vi "Airmar Interpret NMEA Sentence.vi"(11 "NMEA Sentence":string) -> ()   [LabVIEW 2013]
doc: "Interprets the NMEA 0813 sentences that we are using from our Airmar PB200 WeatherStation sensor.\nBy Jaime McCandless\nTODO: finish implementing NMEA sentences"
uses:
  Data/TypeDefs/UTM Location.ctl
  Data/TypeDefs/Notifiers.ctl
  Data/TypeDefs/GPS Sensor Status.ctl
  Data/TypeDefs/Sail Set Suggestions.ctl
  Data/TypeDefs/Rudder Set Suggestions.ctl
  <vilib>/regexp/Match Regular Expression.xnode
panel:
  in  "NotifierReff 2":T1
  in  "UTC Time Zone":i32=-5
  in  "Tab Control":T2(tab)
  out "GPS (GGA) Data":T3
  out "GPS (GLL) Data":T4
  out "GPGSA Data":T5
  out "UTC Time":timestamp
  out "Local Time":timestamp
  out "Lattitude (ddmm.mmmm)":dbl format="%_8g"
  out "Lattitude North/South":string
  out "Longitude (ddmm.mmmm)":dbl format="%_8g"
  out "Longitude East/West":string
  out "Speed over ground (knots)":dbl format="%_3g"
  out "Course over ground (degrees)":dbl format="%_4g"
  out "Magnetic Variation (degrees)":dbl format="%_4g"
  out "Variation East/West":string
  out "GPS (RMC) Data":T6 {"Course over ground (degrees)" format="%#.6g"; "Speed over ground (knots)" format="%#.6g"; "Magnetic Variation (degrees)" format="%#.6g"; "Longitude (ddmm.mmmm)" format="%#.6g"; "Lattitude (ddmm.mmmm)" format="%#.6g"}
  out "GPS Data Valid?":bool
  out "Robot UTM Location":T7 {"North" format="%#_10f"; "East" format="%#_8f"}
  out "GPS (VTG) Data":T8
  out "Heading":dbl
  out "Turn (ROT) Data":T9
  out "Meteorological Data":T10
  out "Relative wind direction":cluster{dbl, "Filtered Value Out":dbl}(graph)
  out "Wind (MWV) Data, Theoretical":T11
  out "Wind (MWV) Data, Relative":T11
  out "Transducer (XDR) B Data":cluster{"Pitch (deg)":dbl, "Roll (deg)":dbl}
  out "Transducer (XDR) A Data":T12
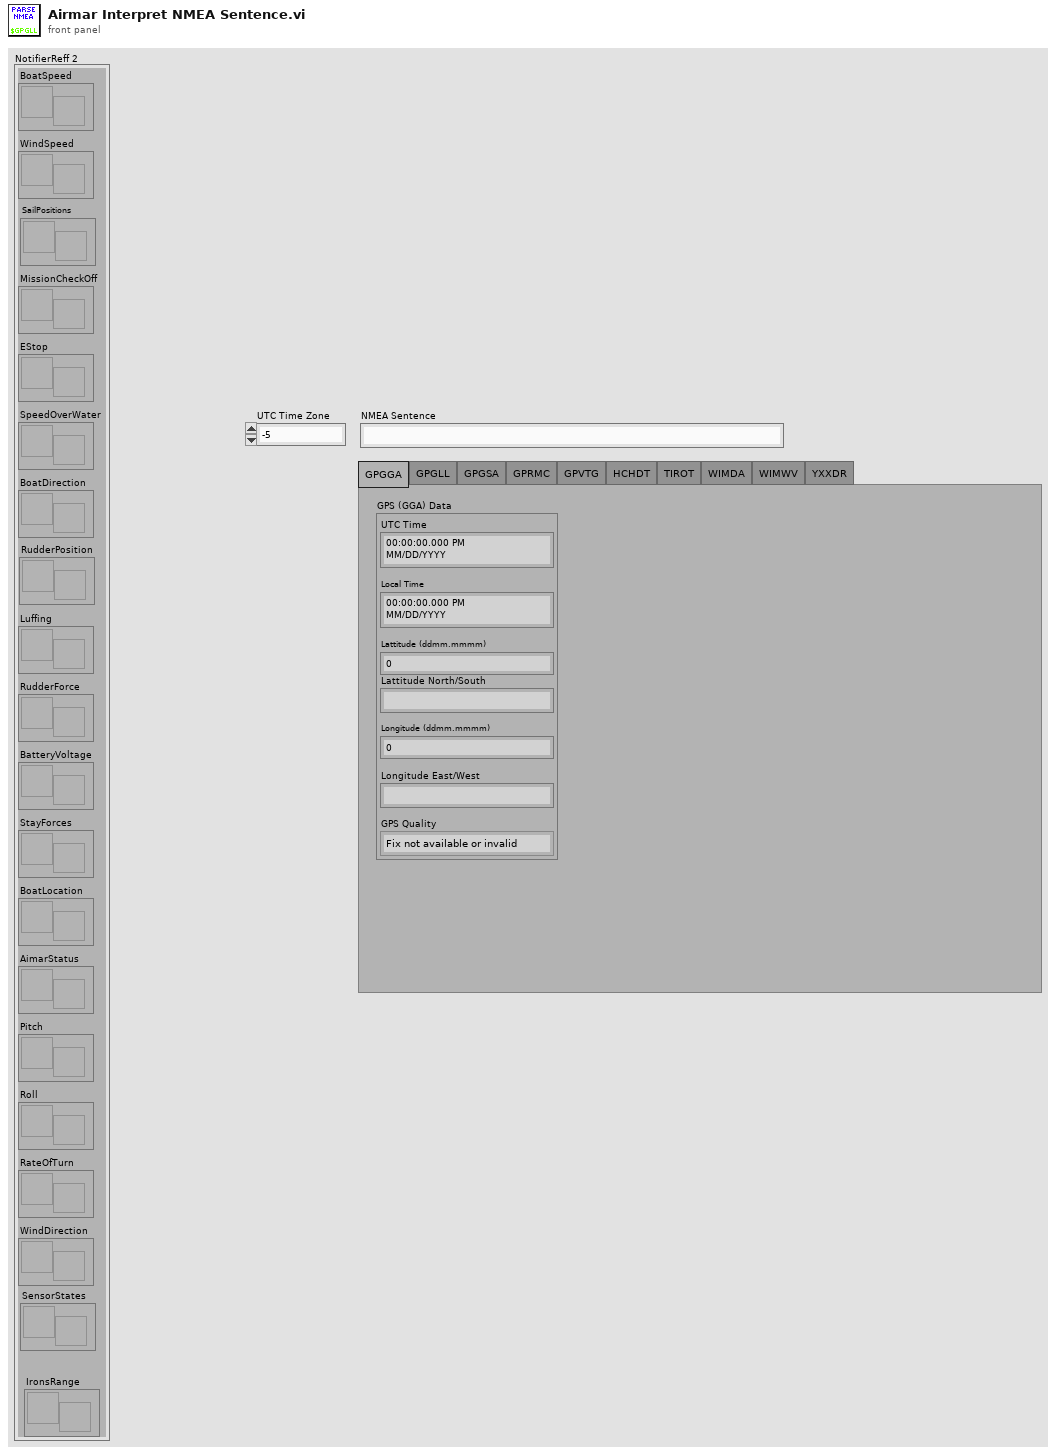
[diagram p1: front panel]
types:
  T1 = typedef "Notifiers.ctl" = cluster{"BoatSpeed":refnum<notifier>, "WindSpeed":refnum<notifier>, "MissionCheckOff":refnum<notifier>, "EStop":refnum<notifier>, "SpeedOverWater":refnum<notifier>, "BoatDirection":refnum<notifier>, "Luffing":refnum<notifier>, "RudderForce":refnum<notifier>, "BatteryVoltage":refnum<notifier>, "StayForces":refnum<notifier>, "BoatLocation":refnum<notifier>, "AimarStatus":refnum<notifier>, "Pitch":refnum<notifier>, "Roll":refnum<notifier>, "RateOfTurn":refnum<notifier>, "WindDirection":refnum<notifier>, "SailPositions":refnum<notifier>, "RudderPosition":refnum<notifier>, "SensorStates":refnum<notifier>, "IronsRange":refnum<notifier>}
  T2 = enum32{"GPGGA", "GPGLL", "GPGSA", "GPRMC", "GPVTG", "HCHDT", "TIROT", "WIMDA", "WIMWV", "YXXDR"}
  T3 = cluster{"UTC Time":timestamp, "Local Time":timestamp, "Lattitude (ddmm.mmmm)":dbl, "Lattitude North/South":string, "Longitude (ddmm.mmmm)":dbl, "Longitude East/West":string, "GPS Quality":enum16{"Fix not available or invalid", "GPS SPS Mode, fix valid", "Differential GPS, SPS Mode, fix valid", "GPS PPS Mode, fix valid", "Real Time Kinematic (RTK)", "Float RTK", "Estimated (dead reckoning) Mode", "Manual Input Mode", "Simulator Mode"}}
  T4 = cluster{"UTC Time":timestamp, "Local Time":timestamp, "Lattitude (ddmm.mmmm)":dbl, "Lattitude North/South":string, "Longitude (ddmm.mmmm)":dbl, "Longitude East/West":string, "GPS Mode":string, "GPS Data Valid?":bool}
  T5 = cluster{"Mode":string, "Fix Strength":i32, "Satellite IDs":i32[], "PDOP":dbl, "HDOP":dbl, "VDOP":dbl}
  T6 = cluster{"UTC Time":timestamp, "Local Time":timestamp, "Lattitude (ddmm.mmmm)":dbl, "Lattitude North/South":string, "Longitude (ddmm.mmmm)":dbl, "Longitude East/West":string, "Magnetic Variation (degrees)":dbl, "Variation East/West":string, "Speed over ground (knots)":dbl, "Course over ground (degrees)":dbl}
  T7 = typedef "UTM Location.ctl" = cluster{"UTM Zone":dbl, "Hemisphere":enum16{"North", "South"}, "East":dbl, "North":dbl}
  T8 = cluster{"Course Over Ground (True)":dbl, "Course Over Ground (Magnetic)":dbl, "Speed Over Ground (Knots)":dbl, "Speed Over Ground (km/hr)":dbl, "GPS Mode":string}
  T9 = cluster{"Rate of Turn (deg/min)":dbl, "Turn Rotation Data Valid?":bool}
  T10 = cluster{"Barometric Pressure (inches of mercury)":dbl, "Barometric Pressure (bars)":dbl, "Air temperature (degC)":dbl, "Relative humidity (%)":dbl, "Wind direction, True (deg)":dbl, "Wind direction, Magnetic (deg)":dbl, "Wind speed (knots)":dbl, "Wind speed (m/s)":dbl}
  T11 = cluster{"Angle relative to boat (deg)":dbl, "Wind Data Valid?":bool, "Wind speed (knots)":dbl, "True (T) or Relative (R)":string}
  T12 = cluster{"Calc. Relative Wind Chill (degC)":dbl, "Calc. Theoretical Wind Chill (degC)":dbl, "Calc. Heat Index (degC)":dbl, "Meas. Barometric Pressure (bars)":dbl}
  T13 = typedef "GPS Sensor Status.ctl" = cluster{"Sensor Connected":bool, "Sensor OK":bool, "GPS Lock":bool, "Sensor Initialized":bool}
  T14 = cluster{"second":i32, "minute":i32, "hour":i32, "day of month":i32, "month":i32, "year":i32, "day of week":i32, "day of year":i32, "is DST":i32}
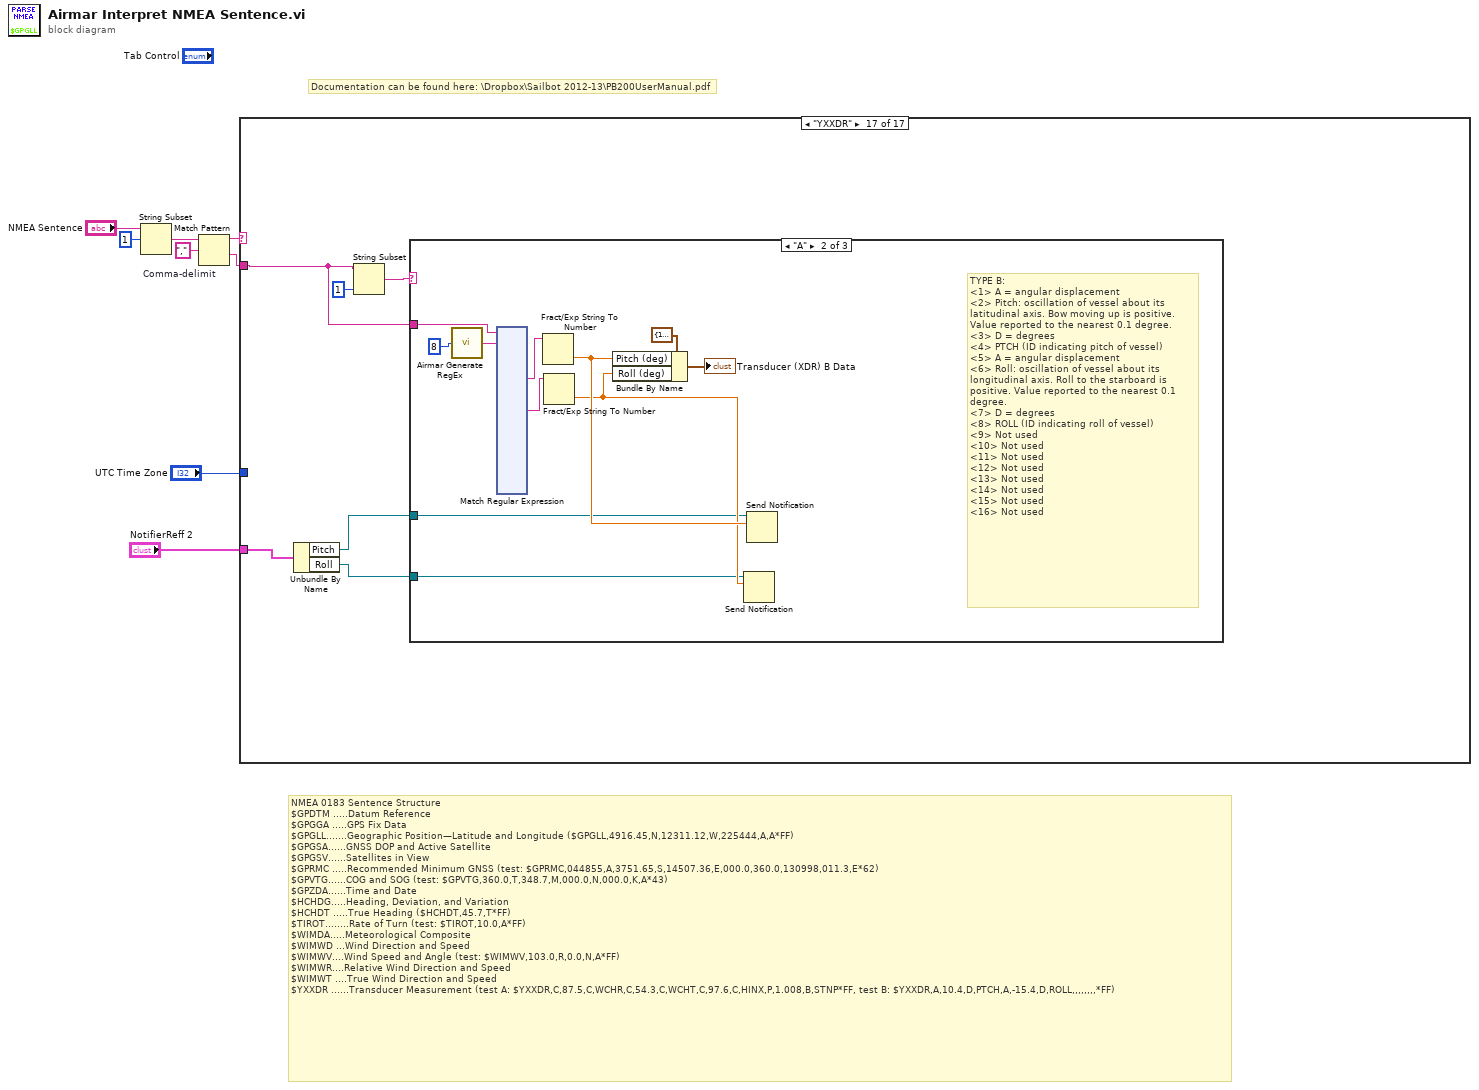
[diagram p0: block diagram]
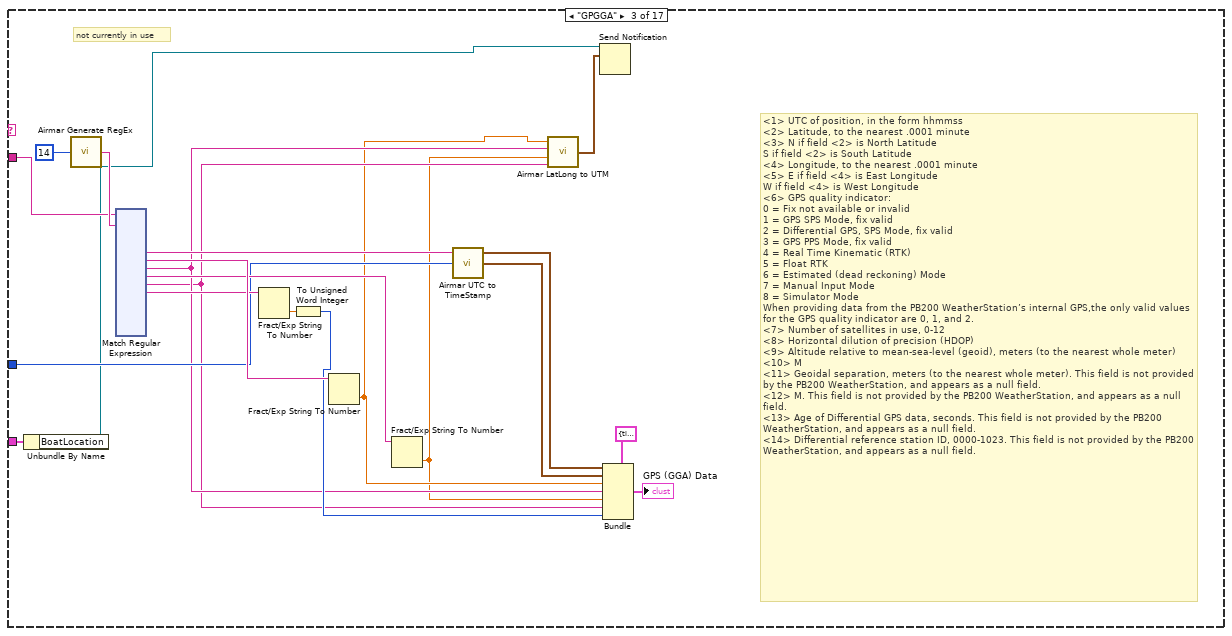
[diagram p4: hidden frame]
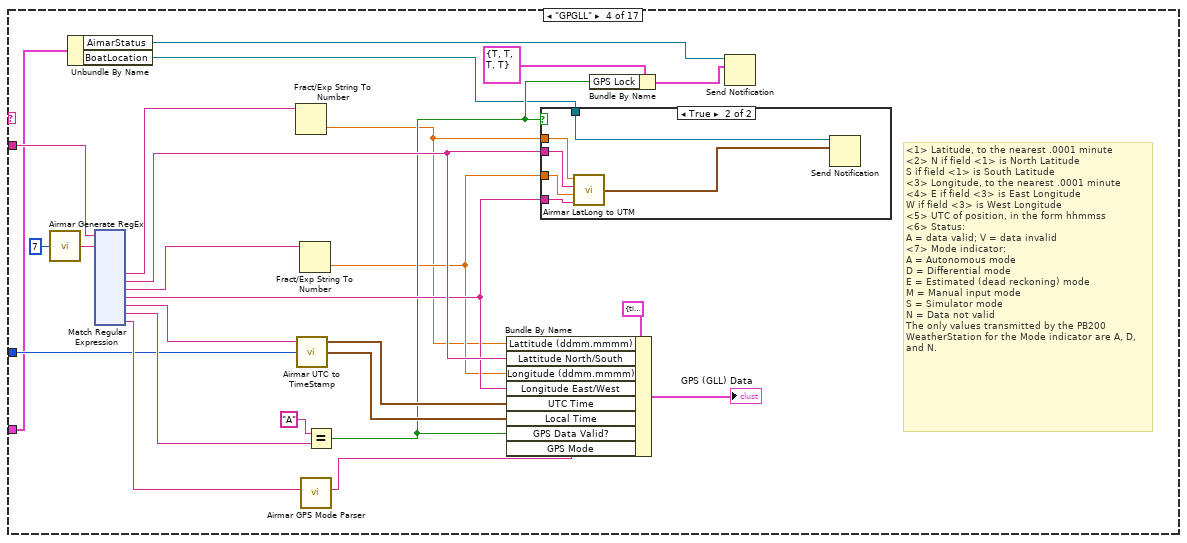
[diagram p5: hidden frame]
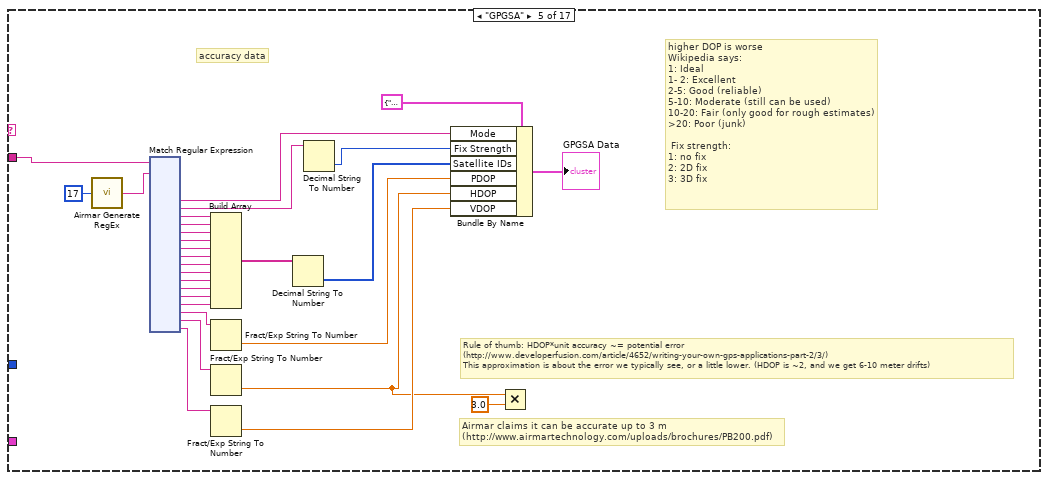
[diagram p7: hidden frame]
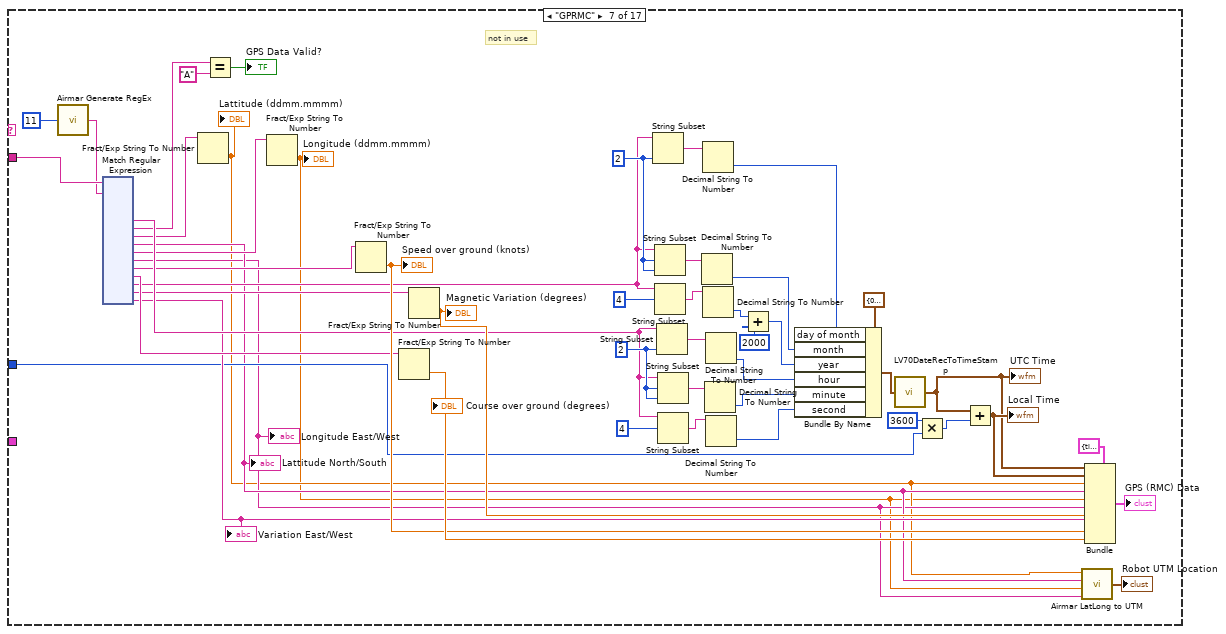
[diagram p9: hidden frame]
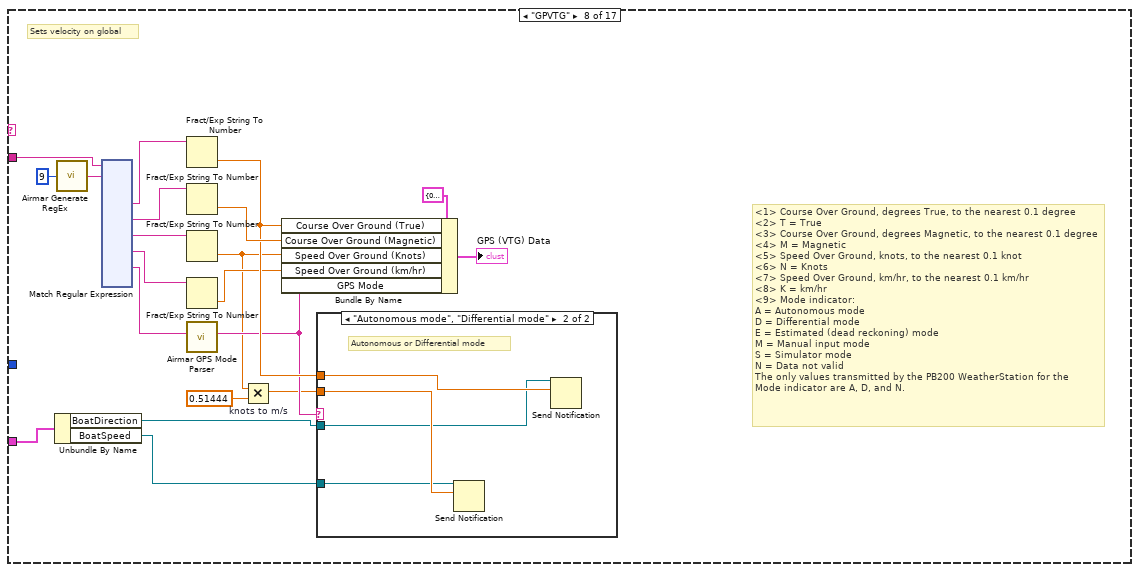
[diagram p10: hidden frame]
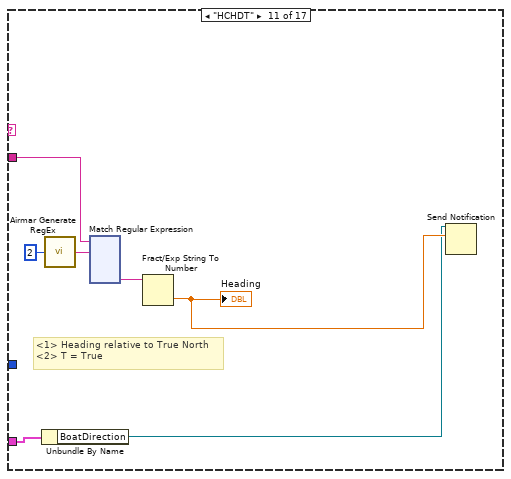
[diagram p14: hidden frame]
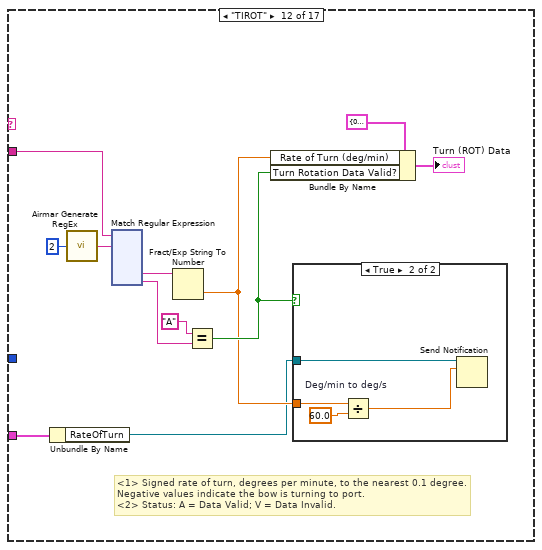
[diagram p15: hidden frame]
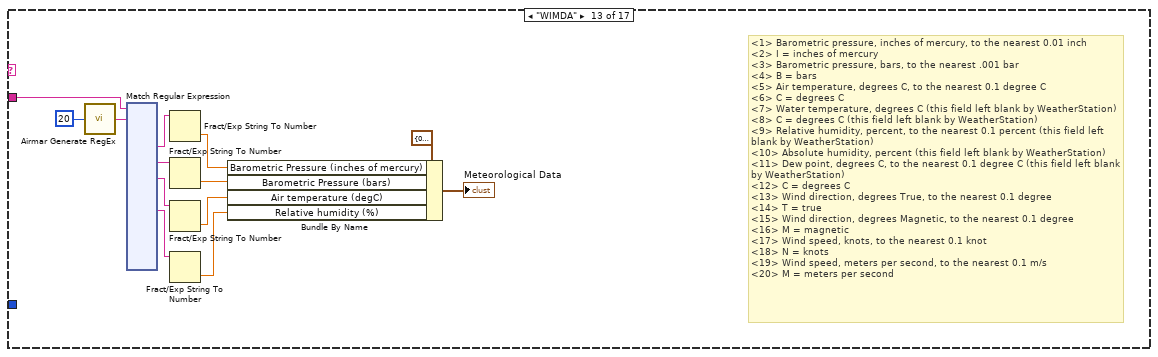
[diagram p17: hidden frame]
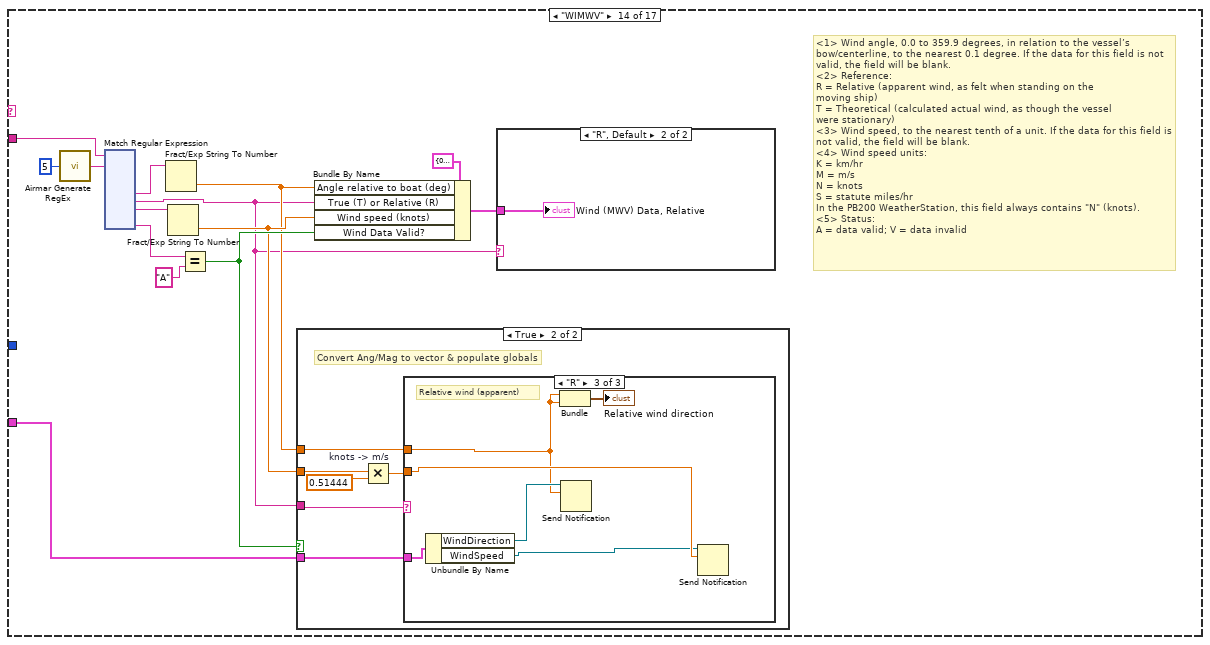
[diagram p18: hidden frame]
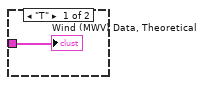
[diagram p19: hidden frame]
diagram:
  # "Documentation can be found here: \\Dropbox\\Sailbot 2012-13\\PB200UserManual.pdf"
  # "NMEA 0183 Sentence Structure\n$GPDTM .....Datum Reference\n$GPGGA .....GPS Fix Data\n$GPGLL.......Geographic Position—Latitude and Longitude ($GPGLL,4916.45,N,12311.12,W,225444,A,A*FF)\n$GPGSA......GNSS DOP and Active Satellite\n$GPGSV......Satellites in View\n$GPRMC .....Recommended Minimum GNSS (test: $GPRMC,044855,A,3751.65,S,14507.36,E,000.0,360.0,130998,011.3,E*62)\n$GPVTG......COG and SOG (test: $GPVTG,360.0,T,348.7,M,000.0,N,000.0,K,A*43)\n$GPZDA......Time and Date\n$HCHDG.....Heading, Deviation, and Variation\n$HCHDT .....True Heading ($HCHDT,45.7,T*FF)\n$TIROT........Rate of Turn (test: $TIROT,10.0,A*FF)\n$WIMDA.....Meteorological Composite\n$WIMWD ...Wind Direction and Speed\n$WIMWV....Wind Speed and Angle (test: $WIMWV,103.0,R,0.0,N,A*FF)\n$WIMWR....Relative Wind Direction and Speed\n$WIMWT ....True Wind Direction and Speed\n$YXXDR ......Transducer Measurement (test A: $YXXDR,C,87.5,C,WCHR,C,54.3,C,WCHT,C,97.6,C,HINX,P,1.008,B,STNP*FF, test B: $YXXDR,A,10.4,D,PTCH,A,-15.4,D,ROLL,,,,,,,,*FF)"
  n1 = String Subset(string="NMEA Sentence", offset (0)=1) -> (substring=w5:string)  [unwired: 1 in]
  n2 = Match Pattern "Comma-delimit"(string=w5, regular expression=",") -> (before substring=w6:string, after substring=w7:string)  [unwired: 1 in, 2 out]
  n3 = case shown="\"YXXDR\"" w6 {
    tunnel: w7 -> [_ _ w27 w172 w331 _ w478 w650 _ _ w784 w908 w1040 w1180 _ _ w1319]
    tunnel: "UTC Time Zone" -> [_ _ w16 w164 _ _ w466 _ _ _ _ _ _ _ _ _ _]
    tunnel: "NotifierReff 2" -> [_ _ w12 w157 _ _ _ w635 _ _ w781 w901 _ w1171 _ _ w1318]
    frame "", Default {
    }
    frame "GPDTM" {
      # "unimplemented"
    }
    frame "GPGGA" {
      # "not currently in use"
      # "<1> UTC of position, in the form hhmmss\n<2> Latitude, to the nearest .0001 minute\n<3> N if field <2> is North Latitude\nS if field <2> is South Latitude\n<4> Longitude, to the nearest .0001 minute\n<5> E if field <4> is East Longitude\nW if field <4> is West Longitude\n<6> GPS quality indicator:\n0 = Fix not available or invalid\n1 = GPS SPS Mode, fix valid\n2 = Differential GPS, SPS Mode, fix valid\n3 = GPS PPS Mode, fix valid\n4 = Real Time Kinematic (RTK)\n5 = Float RTK\n6 = Estimated (dead reckoning) Mode\n7 = Manual Input Mode\n8 = Simulator Mode\nWhen providing data from the PB200 WeatherStation’s internal GPS,the only valid values for the GPS quality indicator are 0, 1, and 2.\n<7> Number of satellites in use, 0-12\n<8> Horizontal dilution of precision (HDOP)\n<9> Altitude relative to mean-sea-level (geoid), meters (to the nearest whole meter)\n<10> M\n<11> Geoidal separation, meters (to the nearest whole meter). This field is not provided by the PB200 WeatherStation, and appears as a null field.\n<12> M. This field is not provided by the PB200 WeatherStation, and appears as a null field.\n<13> Age of Differential GPS data, seconds. This field is not provided by the PB200 WeatherStation, and appears as a null field.\n<14> Differential reference station ID, 0000-1023. This field is not provided by the PB200 WeatherStation, and appears as a null field."
      n4 = Unbundle By Name(w12) -> ("BoatLocation"=w11:refnum<notifier>)
      n5 = call "Airmar Generate RegEx.vi"("# Datums"=14) -> ("RegEx"=w28:string)
      n6 = xnode "Match Regular Expression"("input string"=w27, "regular expression"=w28) -> ("submatch 1"=w19:string, "submatch 2"=w25:string, "submatch 3"=w15:string, "submatch 4"=w24:string, "submatch 5"=w14:string, "submatch 6"=w23:string)  [unwired: 4 in, 10 out]
      n7 = Fract/Exp String To Number(string=w23) -> (number=w22:dbl)  [unwired: 3 in, 1 out]
      n8 = To Unsigned Word Integer(number=w22) -> (unsigned 16bit integer=w21:u16)
      n9 = Fract/Exp String To Number(string=w25) -> (number=w10:dbl)  [unwired: 3 in, 1 out]
      n10 = Fract/Exp String To Number(string=w24) -> (number=w9:dbl)  [unwired: 3 in, 1 out]
      n11 = call "Airmar UTC to TimeStamp.vi"("UTC Time Zone in"=w16, "UTC (hhmmss)"=w19) -> ("Local Time"=w17:timestamp, "UTC Time"=w18:timestamp)  [unwired: 2 in]
      n12 = call "Airmar LatLong to UTM.vi"("East/West"=w14, "Longitude"=w9, "North/South"=w15, "Latitude"=w10) -> ("Robot UTM Location"=w13:T7)
      n13 = Send Notification(notification=w13, notifier=w11) -> ()  [unwired: 1 in, 2 out]
      n14 = Bundle(cluster=T3 {"UTC Time"=timestamp(0 s since 1904-01-01), "Local Time"=timestamp(0 s since 1904-01-01), "Lattitude (ddmm.mmmm)"=0.0, "Lattitude North/South"="", "Longitude (ddmm.mmmm)"=0.0, "Longitude East/West"="", "GPS Quality"=enum."GPS SPS Mode, fix valid"} ("Cluster"), "UTC Time"=w18, "Local Time"=w17, "Lattitude (ddmm.mmmm)"=w10, "Lattitude North/South"=w15, "Longitude (ddmm.mmmm)"=w9, "Longitude East/West"=w14, "GPS Quality"=w21) -> (→"GPS (GGA) Data":T3)
    }
    frame "GPGLL" {
      # "<1> Latitude, to the nearest .0001 minute\n<2> N if field <1> is North Latitude\nS if field <1> is South Latitude\n<3> Longitude, to the nearest .0001 minute\n<4> E if field <3> is East Longitude\nW if field <3> is West Longitude\n<5> UTC of position, in the form hhmmss\n<6> Status:\nA = data valid; V = data invalid\n<7> Mode indicator:\nA = Autonomous mode\nD = Differential mode\nE = Estimated (dead reckoning) mode\nM = Manual input mode\nS = Simulator mode\nN = Data not valid\nThe only values transmitted by the PB200 WeatherStation for the Mode indicator are A, D, and N."
      n15 = call "Airmar Generate RegEx.vi"("# Datums"=7) -> ("RegEx"=w176:string)
      n16 = Unbundle By Name(w157) -> ("AimarStatus"=w153:refnum<notifier>, "BoatLocation"=w156:refnum<notifier>)
      n17 = xnode "Match Regular Expression"("input string"=w172, "regular expression"=w176) -> ("submatch 1"=w175:string, "submatch 2"=w162:string, "submatch 3"=w174:string, "submatch 4"=w161:string, "submatch 5"=w171:string, "submatch 6"=w167:string, "submatch 7"=w173:string)  [unwired: 4 in, 5 out]
      n18 = Fract/Exp String To Number(string=w175) -> (number=w154:dbl)  [unwired: 3 in, 1 out]
      n19 = call "Airmar UTC to TimeStamp.vi"("UTC Time Zone in"=w164, "UTC (hhmmss)"=w171) -> ("Local Time"=w166:timestamp, "UTC Time"=w165:timestamp)  [unwired: 2 in]
      n20 = Fract/Exp String To Number(string=w174) -> (number=w155:dbl)  [unwired: 3 in, 1 out]
      n21 = call "Airmar GPS Mode Parser.vi"("GPS Mode (Char)"=w173) -> ("GPS Mode (Description)"=w169:string)  [unwired: 6 in]
      n22 = Equal?(x="A" ("y"), y=w167) -> (x = y?=w160:bool)
      n23 = Bundle By Name(cluster=T4 {"UTC Time"=timestamp(0 s since 1904-01-01), "Local Time"=timestamp(0 s since 1904-01-01), "Lattitude (ddmm.mmmm)"=0.0, "Lattitude North/South"="", "Longitude (ddmm.mmmm)"=0.0, "Longitude East/West"="", "GPS Mode"="", "GPS Data Valid?"=FALSE} ("Cluster"), "Lattitude (ddmm.mmmm)"=w154, "Lattitude North/South"=w162, "Longitude (ddmm.mmmm)"=w155, "Longitude East/West"=w161, "UTC Time"=w165, "Local Time"=w166, "GPS Data Valid?"=w160, "GPS Mode"=w169) -> (→"GPS (GLL) Data":T4)
      n24 = case shown="True" w160 {
        tunnel: w162 -> [_ w183]
        tunnel: w155 -> [_ w182]
        tunnel: w161 -> [_ w181]
        tunnel: w156 -> [_ w179]
        tunnel: w154 -> [_ w178]
        frame False {
        }
        frame True {
          n25 = call "Airmar LatLong to UTM.vi"("East/West"=w181, "Longitude"=w182, "North/South"=w183, "Latitude"=w178) -> ("Robot UTM Location"=w180:T7)
          n26 = Send Notification(notification=w180, notifier=w179) -> ()  [unwired: 1 in, 2 out]
        }
      }
      n27 = Bundle By Name(cluster=T13 {"Sensor Connected"=TRUE, "Sensor OK"=TRUE, "GPS Lock"=TRUE, "Sensor Initialized"=TRUE} ("input cluster"), "GPS Lock"=w160) -> (w158:T13)
      n28 = Send Notification(notification=w158, notifier=w153) -> ()  [unwired: 1 in, 2 out]
    }
    frame "GPGSA" {
      # "Airmar claims it can be accurate up to 3 m\n(http://www.airmartechnology.com/uploads/brochures/PB200.pdf)"
      # "Rule of thumb: HDOP*unit accuracy ~= potential error\n(http://www.developerfusion.com/article/4652/writing-your-own-gps-applications-part-2/3/)\nThis approximation is about the error we typically see, or a little lower. (HDOP is ~2, and we get 6-10 meter drifts)"
      # "higher DOP is worse\nWikipedia says:\n1: Ideal\n1- 2: Excellent\n2-5: Good (reliable)\n5-10: Moderate (still can be used)\n10-20: Fair (only good for rough estimates)\n>20: Poor (junk)\n\n Fix strength: \n1: no fix\n2: 2D fix\n3: 3D fix"
      # "accuracy data"
      n29 = call "Airmar Generate RegEx.vi"("# Datums"=17) -> ("RegEx"=w330:string)
      n30 = xnode "Match Regular Expression"("input string"=w331, "regular expression"=w330) -> ("submatch 1"=w327:string, "submatch 2"=w326:string, "submatch 3"=w324:string, "submatch 4"=w323:string, "submatch 5"=w322:string, "submatch 6"=w321:string, "submatch 7"=w320:string, "submatch 8"=w319:string, "submatch 9"=w318:string, "submatch 10"=w317:string, "submatch 11"=w316:string, "submatch 12"=w315:string, "submatch 13"=w314:string, "submatch 14"=w313:string, "submatch 15"=w310:string, "submatch 16"=w308:string, "submatch 17"=w307:string)  [unwired: 4 in, 5 out]
      n31 = Build Array(w324, w323, w322, w321, w320, w319, w318, w317, w316, w315, w314, w313) -> (w312:string[])
      n32 = Fract/Exp String To Number(string=w310) -> (number=w309:dbl)  [unwired: 3 in, 1 out]
      n33 = Fract/Exp String To Number(string=w308) -> (number=w304:dbl)  [unwired: 3 in, 1 out]
      n34 = Fract/Exp String To Number(string=w307) -> (number=w306:dbl)  [unwired: 3 in, 1 out]
      n35 = Decimal String To Number(string=w312) -> (number=w311:i32[])  [unwired: 2 in, 1 out]
      n36 = Decimal String To Number(string=w326) -> (number=w325:i32)  [unwired: 2 in, 1 out]
      n37 = Bundle By Name(cluster=T5 {"Mode"="", "Fix Strength"=0, "Satellite IDs"=[], "PDOP"=0.0, "HDOP"=0.0, "VDOP"=0.0} ("GPGSA Data"), "Mode"=w327, "Fix Strength"=w325, "Satellite IDs"=w311, "PDOP"=w309, "HDOP"=w304, "VDOP"=w306) -> (→"GPGSA Data":T5)
      n38 = Multiply(x=w304, y=3.0) -> ()  [unwired: 1 out]
    }
    frame "GPGSV" {
      # "unimplemented"
    }
    frame "GPRMC" {
      w496 = 2 ("length (rest)")
      w486 = 2 ("length (rest)")
      # "not in use"
      n39 = call "Airmar Generate RegEx.vi"("# Datums"=11) -> ("RegEx"=w468:string)
      n40 = xnode "Match Regular Expression"("input string"=w478, "regular expression"=w468) -> ("submatch 1"=w477:string, "submatch 2"=w476:string, "submatch 3"=w475:string, "submatch 4"=w465:string, "submatch 5"=w474:string, "submatch 6"=w464:string, "submatch 7"=w473:string, "submatch 8"=w472:string, "submatch 9"=w471:string, "submatch 10"=w470:string, "submatch 11"=w469:string)  [unwired: 4 in, 5 out]
      "Lattitude North/South" <- w465
      "Longitude East/West" <- w464
      "Variation East/West" <- w469
      n41 = Fract/Exp String To Number(string=w475) -> (number=w462:dbl)  [unwired: 3 in, 1 out]
      "Lattitude (ddmm.mmmm)" <- w462
      n42 = Equal?(x=w476, y="A") -> (x = y?=→"GPS Data Valid?":bool)
      n43 = Fract/Exp String To Number(string=w474) -> (number=w461:dbl)  [unwired: 3 in, 1 out]
      "Longitude (ddmm.mmmm)" <- w461
      n44 = Fract/Exp String To Number(string=w473) -> (number=w506:dbl)  [unwired: 3 in, 1 out]
      "Speed over ground (knots)" <- w506
      n45 = Fract/Exp String To Number(string=w472) -> (number=w507:dbl)  [unwired: 3 in, 1 out]
      "Course over ground (degrees)" <- w507
      n46 = Fract/Exp String To Number(string=w470) -> (number=w505:dbl)  [unwired: 3 in, 1 out]
      "Magnetic Variation (degrees)" <- w505
      n47 = String Subset(string=w471, length (rest)=w496) -> (substring=w497:string)  [unwired: 1 in]
      n48 = String Subset(string=w471, offset (0)=w496, length (rest)=w496) -> (substring=w495:string)
      n49 = String Subset(string=w471, offset (0)=4) -> (substring=w493:string)  [unwired: 1 in]
      n50 = String Subset(string=w477, length (rest)=w486) -> (substring=w482:string)  [unwired: 1 in]
      n51 = String Subset(string=w477, offset (0)=w486, length (rest)=w486) -> (substring=w488:string)
      n52 = String Subset(string=w477, offset (0)=4) -> (substring=w490:string)  [unwired: 1 in]
      n53 = Decimal String To Number(string=w495) -> (number=w499:i32)  [unwired: 2 in, 1 out]
      n54 = Decimal String To Number(string=w497) -> (number=w498:i32)  [unwired: 2 in, 1 out]
      n55 = Decimal String To Number(string=w493) -> (number=w500:i32)  [unwired: 2 in, 1 out]
      n56 = Decimal String To Number(string=w488) -> (number=w487:i32)  [unwired: 2 in, 1 out]
      n57 = Decimal String To Number(string=w482) -> (number=w485:i32)  [unwired: 2 in, 1 out]
      n58 = Decimal String To Number(string=w490) -> (number=w491:i32)  [unwired: 2 in, 1 out]
      n59 = Add(x=w500, y=2000) -> (x+y=w502:i32)
      n60 = Bundle By Name(cluster=T14 {"second"=0, "minute"=0, "hour"=0, "day of month"=0, "month"=0, "year"=0, "day of week"=0, "day of year"=0, "is DST"=0} ("date time rec"), "day of month"=w498, "month"=w499, "year"=w502, "hour"=w485, "minute"=w487, "second"=w491) -> (w483:T14)
      n61 = call <vilib>:"LV70DateRecToTimeStamp.vi"("date time rec"=w483) -> ("Time Stamp"=w503:timestamp)
      "UTC Time" <- w503
      n62 = Multiply(x=3600 ("number"), y=w466) -> (x*y=w467:i32)
      n63 = Add(x=w503, y=w467) -> (x+y=w504:timestamp)
      "Local Time" <- w504
      n64 = call "Airmar LatLong to UTM.vi"("East/West"=w464, "Longitude"=w461, "North/South"=w465, "Latitude"=w462) -> ("Robot UTM Location"=→"Robot UTM Location":T7)
      n65 = Bundle(cluster=T6 {"UTC Time"=timestamp(0 s since 1904-01-01), "Local Time"=timestamp(0 s since 1904-01-01), "Lattitude (ddmm.mmmm)"=0.0, "Lattitude North/South"="", "Longitude (ddmm.mmmm)"=0.0, "Longitude East/West"="", "Magnetic Variation (degrees)"=0.0, "Variation East/West"="", "Speed over ground (knots)"=0.0, "Course over ground (degrees)"=0.0} ("Cluster"), "UTC Time"=w503, "Local Time"=w504, "Lattitude (ddmm.mmmm)"=w462, "Lattitude North/South"=w465, "Longitude (ddmm.mmmm)"=w461, "Longitude East/West"=w464, "Magnetic Variation (degrees)"=w505, "Variation East/West"=w469, "Speed over ground (knots)"=w506, "Course over ground (degrees)"=w507) -> (→"GPS (RMC) Data":T6)
    }
    frame "GPVTG" {
      # "Sets velocity on global"
      # "<1> Course Over Ground, degrees True, to the nearest 0.1 degree\n<2> T = True\n<3> Course Over Ground, degrees Magnetic, to the nearest 0.1 degree\n<4> M = Magnetic\n<5> Speed Over Ground, knots, to the nearest 0.1 knot\n<6> N = Knots\n<7> Speed Over Ground, km/hr, to the nearest 0.1 km/hr\n<8> K = km/hr\n<9> Mode indicator:\nA = Autonomous mode\nD = Differential mode\nE = Estimated (dead reckoning) mode\nM = Manual input mode\nS = Simulator mode\nN = Data not valid\nThe only values transmitted by the PB200 WeatherStation for the\nMode indicator are A, D, and N."
      n66 = Unbundle By Name(w635) -> ("BoatDirection"=w634:refnum<notifier>, "BoatSpeed"=w633:refnum<notifier>)
      n67 = call "Airmar Generate RegEx.vi"("# Datums"=9) -> ("RegEx"=w651:string)
      n68 = xnode "Match Regular Expression"("input string"=w650, "regular expression"=w651) -> ("submatch 1"=w647:string, "submatch 3"=w646:string, "submatch 5"=w644:string, "submatch 7"=w643:string, "submatch 9"=w642:string)  [unwired: 4 in, 11 out]
      n69 = Fract/Exp String To Number(string=w647) -> (number=w641:dbl)  [unwired: 3 in, 1 out]
      n70 = Fract/Exp String To Number(string=w646) -> (number=w645:dbl)  [unwired: 3 in, 1 out]
      n71 = Fract/Exp String To Number(string=w644) -> (number=w638:dbl)  [unwired: 3 in, 1 out]
      n72 = Fract/Exp String To Number(string=w643) -> (number=w640:dbl)  [unwired: 3 in, 1 out]
      n73 = call "Airmar GPS Mode Parser.vi"("GPS Mode (Char)"=w642) -> ("GPS Mode (Description)"=w639:string)  [unwired: 6 in]
      n74 = Multiply "knots to m/s"(x=w638, y=0.51444) -> (x*y=w637:dbl)
      n75 = Bundle By Name(cluster=T8 {"Course Over Ground (True)"=0.0, "Course Over Ground (Magnetic)"=0.0, "Speed Over Ground (Knots)"=0.0, "Speed Over Ground (km/hr)"=0.0, "GPS Mode"=""} ("GPS (VTG) Data 2"), "Course Over Ground (True)"=w641, "Course Over Ground (Magnetic)"=w645, "Speed Over Ground (Knots)"=w638, "Speed Over Ground (km/hr)"=w640, "GPS Mode"=w639) -> (→"GPS (VTG) Data":T8)
      n76 = case shown="\"Autonomous mode\", \"Differential mode\"" w639 {
        tunnel: w641 -> [_ w655]
        tunnel: w637 -> [_ w656]
        tunnel: w634 -> [_ w654]
        tunnel: w633 -> [_ w653]
        frame "Data not valid", Default {
          # "Data not valid"
        }
        frame "Autonomous mode", "Differential mode" {
          # "Autonomous or Differential mode"
          n77 = Send Notification(notification=w656, notifier=w653) -> ()  [unwired: 1 in, 2 out]
          n78 = Send Notification(notification=w655, notifier=w654) -> ()  [unwired: 1 in, 2 out]
        }
      }
    }
    frame "GPZDA" {
      # "<1> UTC time of day, in the form hhmmss\n<2> UTC day, 01 to 31\n<3> UTC month, 01 to 12\n<4> UTC year (four digits, e.g. 2006)\n<5> Local time zone hours, 00 to +/-13 hrs\n<6> Local time zone minutes, 00 to +59"
    }
    frame "HCHDG " {
      # "<1> Magnetic sensor heading, degrees, to the nearest 0.1 degree.\n<2> Magnetic deviation, degrees east or west, to the nearest 0.1 degree.\n<3> E if field <2> is degrees East\nW if field <2> is degrees West\n<4> Magnetic variation, degrees east or west, to the nearest 0.1 degree.\n<5> E if field <4> is degrees East\nW if field <4> is degrees West"
    }
    frame "HCHDT" {
      # "<1> Heading relative to True North\n<2> T = True"
      n79 = Unbundle By Name(w781) -> ("BoatDirection"=w780:refnum<notifier>)
      n80 = call "Airmar Generate RegEx.vi"("# Datums"=2) -> ("RegEx"=w785:string)
      n81 = xnode "Match Regular Expression"("input string"=w784, "regular expression"=w785) -> ("submatch 1"=w783:string)  [unwired: 4 in, 5 out]
      n82 = Fract/Exp String To Number(string=w783) -> (number=w782:dbl)  [unwired: 3 in, 1 out]
      "Heading" <- w782
      n83 = Send Notification(notification=w782, notifier=w780) -> ()  [unwired: 1 in, 2 out]
    }
    frame "TIROT" {
      # "<1> Signed rate of turn, degrees per minute, to the nearest 0.1 degree.\nNegative values indicate the bow is turning to port.\n<2> Status: A = Data Valid; V = Data Invalid."
      n84 = Unbundle By Name(w901) -> ("RateOfTurn"=w900:refnum<notifier>)
      n85 = call "Airmar Generate RegEx.vi"("# Datums"=2) -> ("RegEx"=w910:string)
      n86 = xnode "Match Regular Expression"("input string"=w908, "regular expression"=w910) -> ("submatch 1"=w909:string, "submatch 2"=w904:string)  [unwired: 4 in, 5 out]
      n87 = Fract/Exp String To Number(string=w909) -> (number=w902:dbl)  [unwired: 3 in, 1 out]
      n88 = Equal?(x="A" ("y"), y=w904) -> (x = y?=w903:bool)
      n89 = Bundle By Name(cluster=T9 {"Rate of Turn (deg/min)"=0.0, "Turn Rotation Data Valid?"=TRUE} ("Turn (ROT) Data 2"), "Rate of Turn (deg/min)"=w902, "Turn Rotation Data Valid?"=w903) -> (→"Turn (ROT) Data":T9)
      n90 = case shown="True" w903 {
        tunnel: w902 -> [_ w915]
        tunnel: w900 -> [_ w912]
        frame False {
        }
        frame True {
          n91 = Divide "Deg/min to deg/s"(x=w915, y=60.0) -> (x/y=w913:dbl)
          n92 = Send Notification(notification=w913, notifier=w912) -> ()  [unwired: 1 in, 2 out]
        }
      }
    }
    frame "WIMDA" {
      # "<1> Barometric pressure, inches of mercury, to the nearest 0.01 inch\n<2> I = inches of mercury\n<3> Barometric pressure, bars, to the nearest .001 bar\n<4> B = bars\n<5> Air temperature, degrees C, to the nearest 0.1 degree C\n<6> C = degrees C\n<7> Water temperature, degrees C (this field left blank by WeatherStation)\n<8> C = degrees C (this field left blank by WeatherStation)\n<9> Relative humidity, percent, to the nearest 0.1 percent (this field left\nblank by WeatherStation)\n<10> Absolute humidity, percent (this field left blank by WeatherStation)\n<11> Dew point, degrees C, to the nearest 0.1 degree C (this field left blank\nby WeatherStation)\n<12> C = degrees C\n<13> Wind direction, degrees True, to the nearest 0.1 degree\n<14> T = true\n<15> Wind direction, degrees Magnetic, to the nearest 0.1 degree\n<16> M = magnetic\n<17> Wind speed, knots, to the nearest 0.1 knot\n<18> N = knots\n<19> Wind speed, meters per second, to the nearest 0.1 m/s\n<20> M = meters per second"
      n93 = call "Airmar Generate RegEx.vi"("# Datums"=20) -> ("RegEx"=w1041:string)
      n94 = xnode "Match Regular Expression"("input string"=w1040, "regular expression"=w1041) -> ("submatch 1"=w1034:string, "submatch 3"=w1033:string, "submatch 5"=w1032:string, "submatch 9"=w1031:string)  [unwired: 4 in, 17 out]
      n95 = Fract/Exp String To Number(string=w1034) -> (number=w1038:dbl)  [unwired: 3 in, 1 out]
      n96 = Fract/Exp String To Number(string=w1033) -> (number=w1037:dbl)  [unwired: 3 in, 1 out]
      n97 = Fract/Exp String To Number(string=w1032) -> (number=w1036:dbl)  [unwired: 3 in, 1 out]
      n98 = Fract/Exp String To Number(string=w1031) -> (number=w1035:dbl)  [unwired: 3 in, 1 out]
      n99 = Bundle By Name(cluster=T10 {"Barometric Pressure (inches of mercury)"=0.0, "Barometric Pressure (bars)"=0.0, "Air temperature (degC)"=0.0, "Relative humidity (%)"=0.0, "Wind direction, True (deg)"=0.0, "Wind direction, Magnetic (deg)"=0.0, "Wind speed (knots)"=0.0, "Wind speed (m/s)"=0.0} ("Meteorological Data"), "Barometric Pressure (inches of mercury)"=w1038, "Barometric Pressure (bars)"=w1037, "Air temperature (degC)"=w1036, "Relative humidity (%)"=w1035) -> (→"Meteorological Data":T10)
    }
    frame "WIMWV" {
      # "<1> Wind angle, 0.0 to 359.9 degrees, in relation to the vessel’s\nbow/centerline, to the nearest 0.1 degree. If the data for this field is not\nvalid, the field will be blank.\n<2> Reference:\nR = Relative (apparent wind, as felt when standing on the\nmoving ship)\nT = Theoretical (calculated actual wind, as though the vessel\nwere stationary)\n<3> Wind speed, to the nearest tenth of a unit. If the data for this field is\nnot valid, the field will be blank.\n<4> Wind speed units:\nK = km/hr\nM = m/s\nN = knots\nS = statute miles/hr\nIn the PB200 WeatherStation, this field always contains \"N\" (knots).\n<5> Status:\nA = data valid; V = data invalid"
      n100 = call "Airmar Generate RegEx.vi"("# Datums"=5) -> ("RegEx"=w1183:string)
      n101 = xnode "Match Regular Expression"("input string"=w1180, "regular expression"=w1183) -> ("submatch 1"=w1182:string, "submatch 2"=w1172:string, "submatch 3"=w1177:string, "submatch 5"=w1176:string)  [unwired: 4 in, 6 out]
      n102 = Fract/Exp String To Number(string=w1182) -> (number=w1173:dbl)  [unwired: 3 in, 1 out]
      n103 = Fract/Exp String To Number(string=w1177) -> (number=w1174:dbl)  [unwired: 3 in, 1 out]
      n104 = Equal?(x=w1176, y="A") -> (x = y?=w1175:bool)
      n105 = case shown="True" w1175 {
        tunnel: w1174 -> [_ w1189]
        tunnel: w1173 -> [_ w1192]
        tunnel: w1172 -> [_ w1191]
        tunnel: w1171 -> [_ w1187]
        frame False {
        }
        frame True {
          # "Convert Ang/Mag to vector & populate globals"
          n106 = Multiply "knots -> m/s"(x=w1189, y=0.51444) -> (x*y=w1190:dbl)
          n107 = case shown="\"R\"" w1191 {
            tunnel: w1190 -> [_ _ w1196]
            tunnel: w1192 -> [_ _ w1193]
            tunnel: w1187 -> [_ _ w1197]
            frame "", Default {
            }
            frame "T" {
              # "Theoretical wind (absolute)"
            }
            frame "R" {
              # "Relative wind (apparent)"
              n108 = Unbundle By Name(w1197) -> ("WindDirection"=w1194:refnum<notifier>, "WindSpeed"=w1195:refnum<notifier>)
              n109 = Bundle(w1193, w1193) -> (→"Relative wind direction":cluster{dbl, dbl})  [unwired: 1 in]
              n110 = Send Notification(notification=w1193, notifier=w1194) -> ()  [unwired: 1 in, 2 out]
              n111 = Send Notification(notification=w1196, notifier=w1195) -> ()  [unwired: 1 in, 2 out]
            }
          }
        }
      }
      n112 = Bundle By Name(cluster=T11 {"Angle relative to boat (deg)"=0.0, "Wind Data Valid?"=TRUE, "Wind speed (knots)"=0.0, "True (T) or Relative (R)"=""} ("Wind (MWV) Data 2"), "Angle relative to boat (deg)"=w1173, "True (T) or Relative (R)"=w1172, "Wind speed (knots)"=w1174, "Wind Data Valid?"=w1175) -> (w1179:T11)
      n113 = case shown="\"R\", Default" w1172 {
        tunnel: w1179 -> [w1185 w1186]
        frame "T" {
          "Wind (MWV) Data, Theoretical" <- w1185
        }
        frame "R", Default {
          "Wind (MWV) Data, Relative" <- w1186
        }
      }
    }
    frame "WIMWR" {
    }
    frame "WIMWT" {
    }
    frame "YXXDR" {
      n114 = Unbundle By Name(w1318) -> ("Pitch"=w1317:refnum<notifier>, "Roll"=w1316:refnum<notifier>)
      n115 = String Subset(string=w1319, length (rest)=1 ("length (rest)")) -> (substring=w1320:string)  [unwired: 1 in]
      n116 = case shown="\"A\"" w1320 {
        tunnel: w1319 -> [_ w1326 w1461]
        tunnel: w1317 -> [_ w1323 _]
        tunnel: w1316 -> [_ w1322 _]
        frame "", Default {
        }
        frame "A" {
          # "TYPE B:\n<1> A = angular displacement\n<2> Pitch: oscillation of vessel about its latitudinal axis. Bow moving up is positive. Value reported to the nearest 0.1 degree.\n<3> D = degrees\n<4> PTCH (ID indicating pitch of vessel)\n<5> A = angular displacement\n<6> Roll: oscillation of vessel about its longitudinal axis. Roll to the starboard is positive. Value reported to the nearest 0.1 degree.\n<7> D = degrees\n<8> ROLL (ID indicating roll of vessel)\n<9> Not used\n<10> Not used\n<11> Not used\n<12> Not used\n<13> Not used\n<14> Not used\n<15> Not used\n<16> Not used"
          n117 = call "Airmar Generate RegEx.vi"("# Datums"=8) -> ("RegEx"=w1330:string)
          n118 = xnode "Match Regular Expression"("input string"=w1326, "regular expression"=w1330) -> ("submatch 2"=w1328:string, "submatch 6"=w1327:string)  [unwired: 4 in, 19 out]
          n119 = Fract/Exp String To Number(string=w1328) -> (number=w1325:dbl)  [unwired: 3 in, 1 out]
          n120 = Fract/Exp String To Number(string=w1327) -> (number=w1324:dbl)  [unwired: 3 in, 1 out]
          n121 = Bundle By Name(cluster=cluster{"Pitch (deg)":dbl, "Roll (deg)":dbl} {"Pitch (deg)"=103.0, "Roll (deg)"=103.0} ("Transducer (XDR) B Data 2"), "Pitch (deg)"=w1325, "Roll (deg)"=w1324) -> (→"Transducer (XDR) B Data":cluster{"Pitch (deg)":dbl, "Roll (deg)":dbl})
          n122 = Send Notification(notification=w1324, notifier=w1322) -> ()  [unwired: 1 in, 2 out]
          n123 = Send Notification(notification=w1325, notifier=w1323) -> ()  [unwired: 1 in, 2 out]
        }
        frame "C" {
          # "TYPE A:\n<1> C = temperature\n<2> Calculated “relative” wind chill temperature, degrees Celsius, to the nearest 0.1 degree\n<3> C = degrees C\n<4> WCHR (ID indicating relative wind chill)\n<5> C = temperature\n<6> Calculated “theoretical” wind chill temperature, degrees Celsius, to the nearest 0.1 degree\n<7> C = degrees C\n<8> WCHT (ID indicating theoretical wind chill)\n<9> C = temperature\n<10> Calculated heat index, degrees Celsius, to the nearest 0.1 degree (this field left blank by WeatherStation)\n<11> C = degrees C\n<12> HINX (ID indicating heat index)\n<13> P = pressure\n<14> Actual measured barometric pressure, or \"station pressure\", bars, to the nearest 0.001 bar\n<15> B = bars\n<16> STNP (ID indicating station pressure)"
          n124 = call "Airmar Generate RegEx.vi"("# Datums"=16) -> ("RegEx"=w1467:string)
          n125 = xnode "Match Regular Expression"("input string"=w1461, "regular expression"=w1467) -> ("submatch 2"=w1465:string, "submatch 6"=w1464:string, "submatch 10"=w1463:string, "submatch 14"=w1462:string)  [unwired: 4 in, 17 out]
          n126 = Fract/Exp String To Number(string=w1465) -> (number=w1471:dbl)  [unwired: 3 in, 1 out]
          n127 = Fract/Exp String To Number(string=w1464) -> (number=w1470:dbl)  [unwired: 3 in, 1 out]
          n128 = Fract/Exp String To Number(string=w1463) -> (number=w1469:dbl)  [unwired: 3 in, 1 out]
          n129 = Fract/Exp String To Number(string=w1462) -> (number=w1468:dbl)  [unwired: 3 in, 1 out]
          n130 = Bundle By Name(cluster=T12 {"Calc. Relative Wind Chill (degC)"=0.0, "Calc. Theoretical Wind Chill (degC)"=0.0, "Calc. Heat Index (degC)"=0.0, "Meas. Barometric Pressure (bars)"=0.0} ("Transducer (XDR) A Data 2"), "Calc. Relative Wind Chill (degC)"=w1471, "Calc. Theoretical Wind Chill (degC)"=w1470, "Calc. Heat Index (degC)"=w1469, "Meas. Barometric Pressure (bars)"=w1468) -> (→"Transducer (XDR) A Data":T12)
        }
      }
    }
  }
